vi "Create Subscriber.vi"(8 "error in (no error)":errorcluster, 9 "Default Value":dbl, 10 "Name":string, 11 "RTFIFODouble in":refnum<class "CIFTag.lvclass">) -> (0 "error out":errorcluster, 3 "RTFIFODouble out":refnum<class "CIFTag.lvclass">)   [LabVIEW 2021, in "CIFTag.lvclass"]
uses:
  CIFTag.lvclass
  D:/dev/CIF-LVCore/src/CIFUtilities/CIFChannels/CIFChannels.lvclass
  CIFUtilities/CIFChannels/Typedef/Direction.ctl
  CIFUtilities/CIFChannels/Typedef/Disconnect Behavior.ctl
  CIFUtilities/CIFChannels/CIFChannels.lvclass/CIFChannels.ctl
  CIFTag.lvclass/CIFTag.ctl
  CIFUtilities/CIFChannels/Write Channel Class.vi
  CIFUtilities/CIFChannels/Accessors/Write Channel State.vi
  CIFUtilities/CIFChannels/Accessors/Write Direction.vi
  CIFUtilities/CIFChannels/Accessors/Write Disconnect Behavior.vi
  CIFUtilities/CIFChannels/Accessors/Write Name.vi
  CIFUtilities/CIFChannels/Accessors/Write Stored Data.vi
  <vilib>/Utility/LVClass/Get LV Class Name.vi
  CIFUtilities/CIFChannels/CIFChannels.lvclass
  D:/dev/CIF-LVCore/src/Channels/CIFChannel/CIFTag.lvclass
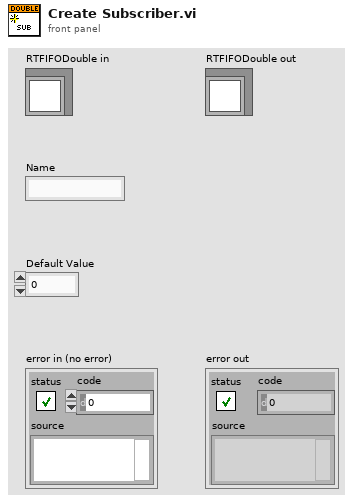
[diagram p1: front panel]
types:
  T1 = typedef "CIFChannels.lvclass/Disconnect Behavior.ctl" = enum16{"Default value", "Last value", "Error with default"}
  T2 = typedef "CIFChannels.lvclass/Direction.ctl" = enum16{"Publisher", "Subscriber"}
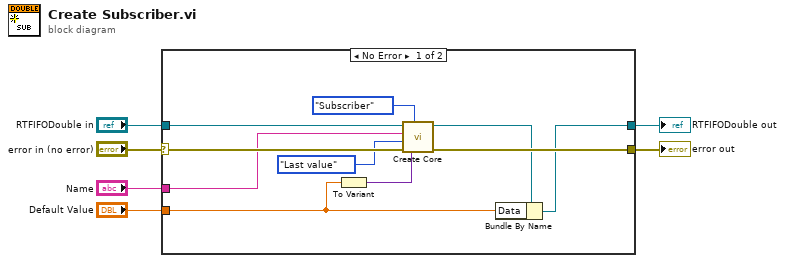
[diagram p0: block diagram]
diagram:
  n1 = case shown="No Error" "error in (no error)" {
    selector: "error in (no error)" -> [w14 w18]
    tunnel: [w10 w18] -> w5
    tunnel: [w7 w17] -> w3
    tunnel: "RTFIFODouble in" -> [w16 w17]
    tunnel: "Name" -> [w11 _]
    tunnel: "Default Value" -> [w8 _]
    frame No Error {
      n2 = To Variant(anything=w8) -> (Variant=w12:variant)
      n3 = call "Create Core.vi"("Stored Data"=w12, "Direction"=Direction."Subscriber", "error in (no error)"=w14, "Disconnect Behavior"=Disconnect_Behavior."Last value", "Name"=w11, "CIFChannels in"=w16) -> ("error out"=w10:errorcluster, "CIFChannels in"=w9:refnum<class "CIFTag.lvclass">)  [unwired: 4 in]
      n4 = Bundle By Name(cluster=w9, "Data"=w8) -> (w7:refnum<class "CIFTag.lvclass">)
    }
    frame Error {
    }
  }
  "error out" <- w5
  "RTFIFODouble out" <- w3
